vi "Sistema de ventilación_sin_entrada.vi"() -> ()   [LabVIEW 2023]
panel:
  out "?":bool
  out "?":bool
  out "?":bool
  out "?":bool
  out "?":bool
  out "?":bool
  out "?":bool
  out "?":bool
  out "?":bool
  out "?":bool
  out "?":bool
  out "?":bool
  out "?":bool
  out "?":bool
  out "?":bool
  out "?":bool
  out "?":bool
  out "?":bool
  in  "Ventilador":bool
  out "Filtro de Calor":bool
  out "Filtro de Aire":bool
  in  "Cluster ppm":cluster{"Gain K [m/mA]":dbl, "Zero u0 [mA]":dbl}
  in  "u [mA] ppm":dbl(slide) scale=0.0..16.0
  out "?":dbl(knob) scale=0.0..1800.0
  out "Temperatura":dbl(slide) scale=0.0..60.0
  out "t [sec]":dbl
  out "Iteration No":i32
  in  "Cluster Temp":cluster{"Gain K [m/mA]":dbl, "Zero u0 [mA]":dbl}
  in  "?":bool
  out "VI is running?":bool caption="ON/OFF"
  in  "u [mA] °C":dbl(slide) scale=0.0..16.0
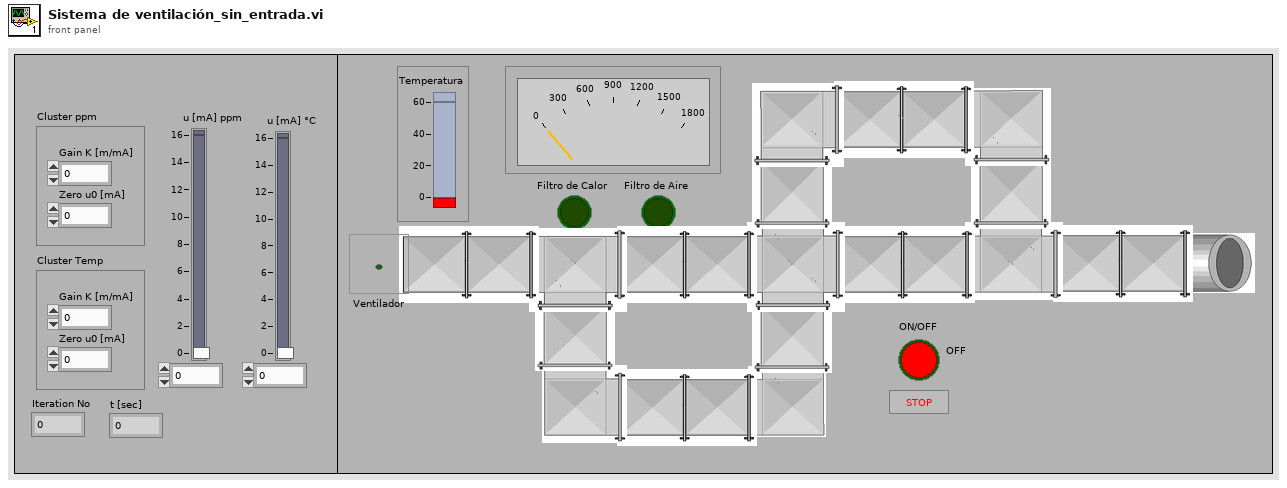
[diagram p1: front panel]
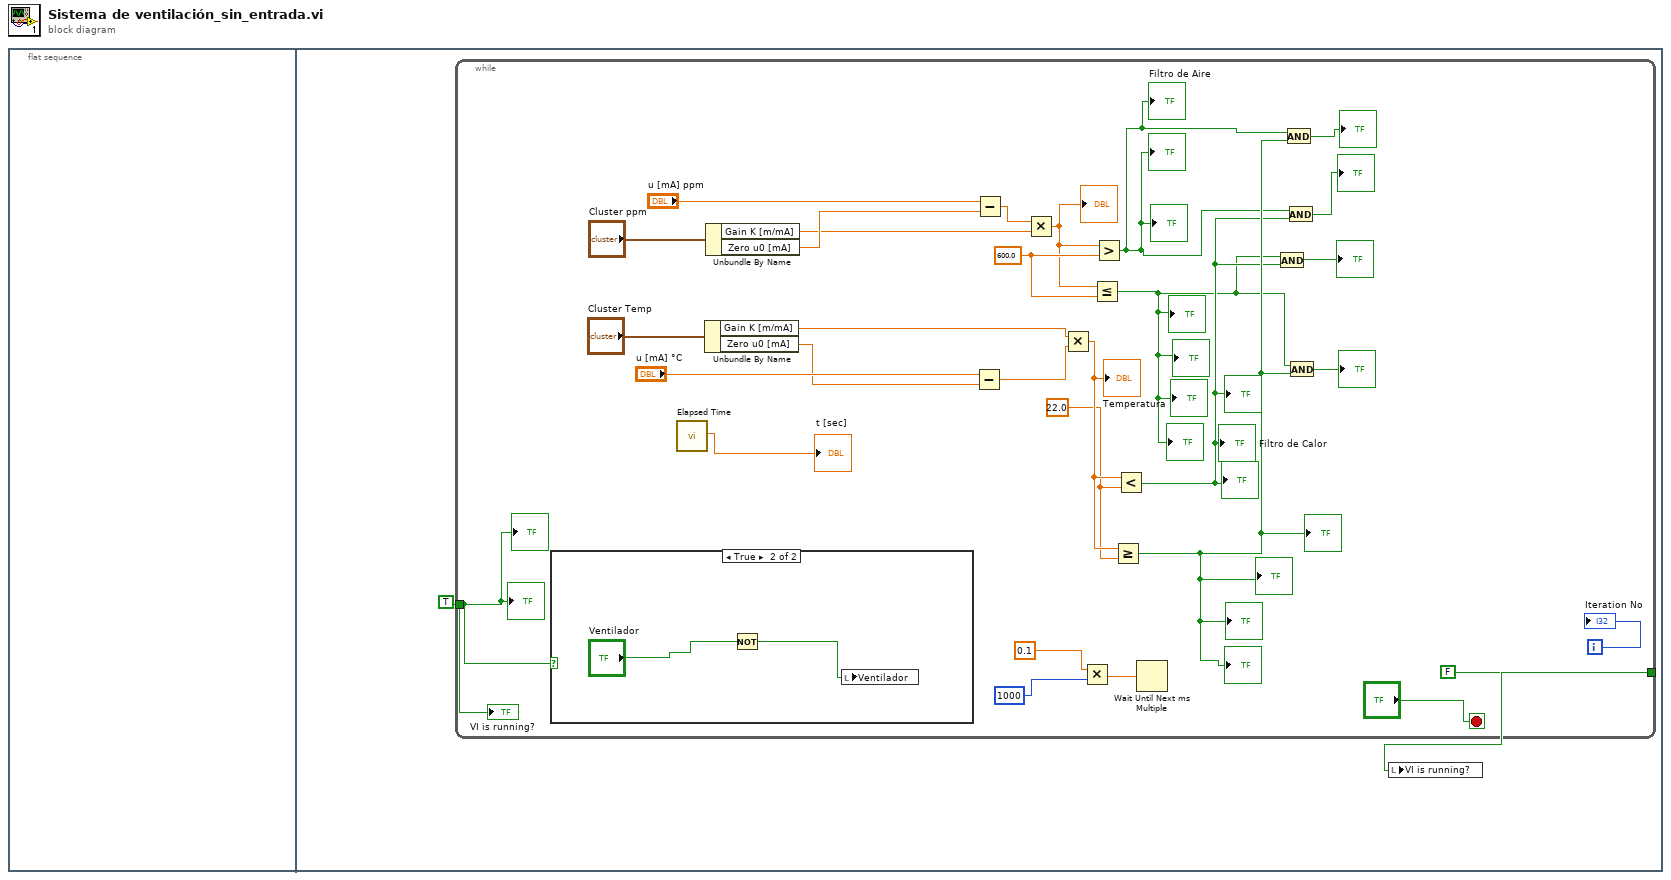
[diagram p0: block diagram]
diagram:
  n1 = flat-sequence {
    frame #0 {
    }
    frame #1 {
      n2 = while {
        tunnel: [FALSE] -> w1
        tunnel: TRUE -> [w10]
        i -> [w24]
        stop <- "?" stop-if-true
        w15 = 600.0
        w12 = 22.0
        n3 = case shown="True" w10 {
          frame False {
          }
          frame True {
            n4 = Not(x="Ventilador") -> (.not. x?=w33:bool)
            n5 = local write "Ventilador"(w33) -> ()
          }
        }
        n6 = call "Elapsed Time"() -> ("Elapsed Time (s)"=→"t [sec]":dbl)  [unwired: 12 in, 7 out]
        n7 = Unbundle By Name "Unbundle By Name"("Cluster Temp") -> ("Gain K [m/mA]"=w16:dbl, "Zero u0 [mA]"=w18:dbl)
        n8 = Unbundle By Name "Unbundle By Name"("Cluster ppm") -> ("Gain K [m/mA]"=w17:dbl, "Zero u0 [mA]"=w19:dbl)
        n9 = Subtract(x="u [mA] °C", y=w18) -> (x-y=w31:dbl)
        n10 = Subtract(x="u [mA] ppm", y=w19) -> (x-y=w21:dbl)
        n11 = Multiply(x=w21, y=w17) -> (x*y=w14:dbl)
        "?" <- w14
        n12 = Multiply(x=w16, y=w31) -> (x*y=w13:dbl)
        "Temperatura" <- w13
        n13 = Multiply(x=0.1, y=1000) -> (x*y=w27:dbl)
        n14 = Less Or Equal?(x=w14, y=w15) -> (x <= y?=w4:bool)
        "?" <- w4
        "?" <- w4
        "?" <- w4
        "?" <- w4
        n15 = Greater?(x=w14, y=w15) -> (0:w8:bool)
        "Filtro de Aire" <- w8
        "?" <- w8
        "?" <- w8
        n16 = Greater Or Equal?(x=w13, y=w12) -> (x >= y?=w9:bool)
        "?" <- w9
        "?" <- w9
        "?" <- w9
        "?" <- w9
        n17 = Less?(x=w13, y=w12) -> (x < y?=w7:bool)
        "Filtro de Calor" <- w7
        "?" <- w7
        "?" <- w7
        n18 = Wait Until Next ms Multiple(millisecond multiple=w27) -> ()  [unwired: 1 out]
        n19 = And(x=w4, y=w7) -> (x .and. y?=→"?":bool)
        n20 = And(x=w8, y=w9) -> (x .and. y?=→"?":bool)
        n21 = And(x=w8, y=w7) -> (x .and. y?=→"?":bool)
        n22 = And(x=w4, y=w9) -> (x .and. y?=→"?":bool)
        "VI is running?" <- w10
        "Iteration No" <- w24
        "?" <- w10
        "?" <- w10
      }
      n23 = local write "VI is running?"(w1) -> ()
    }
  }
